vi "new_coating.vi"(0 "Coating":i32(listbox)) -> (1 "Recipe":string[](array[string]), 2 "Path Array":string[](array[string]))   [LabVIEW 2009]
panel:
  in  "Coating Name :":string
  in  "Recipe List":i32(listbox)
  in  "Move down":bool
  in  "Move up":bool
  out "error out":errorcluster
  in  "delete":bool
  in  "cancel":bool
  in  "ok":bool
  in  "Add Recipe":bool
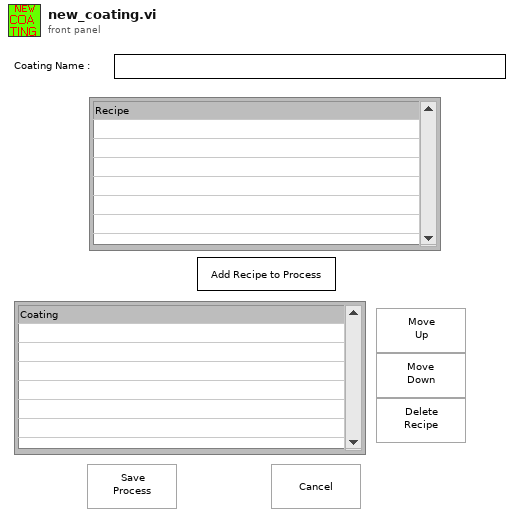
[diagram p1: front panel]
types:
  T1 = enum16{"open", "replace", "create", "open or create", "replace or create", "replace or create with confirmation"}
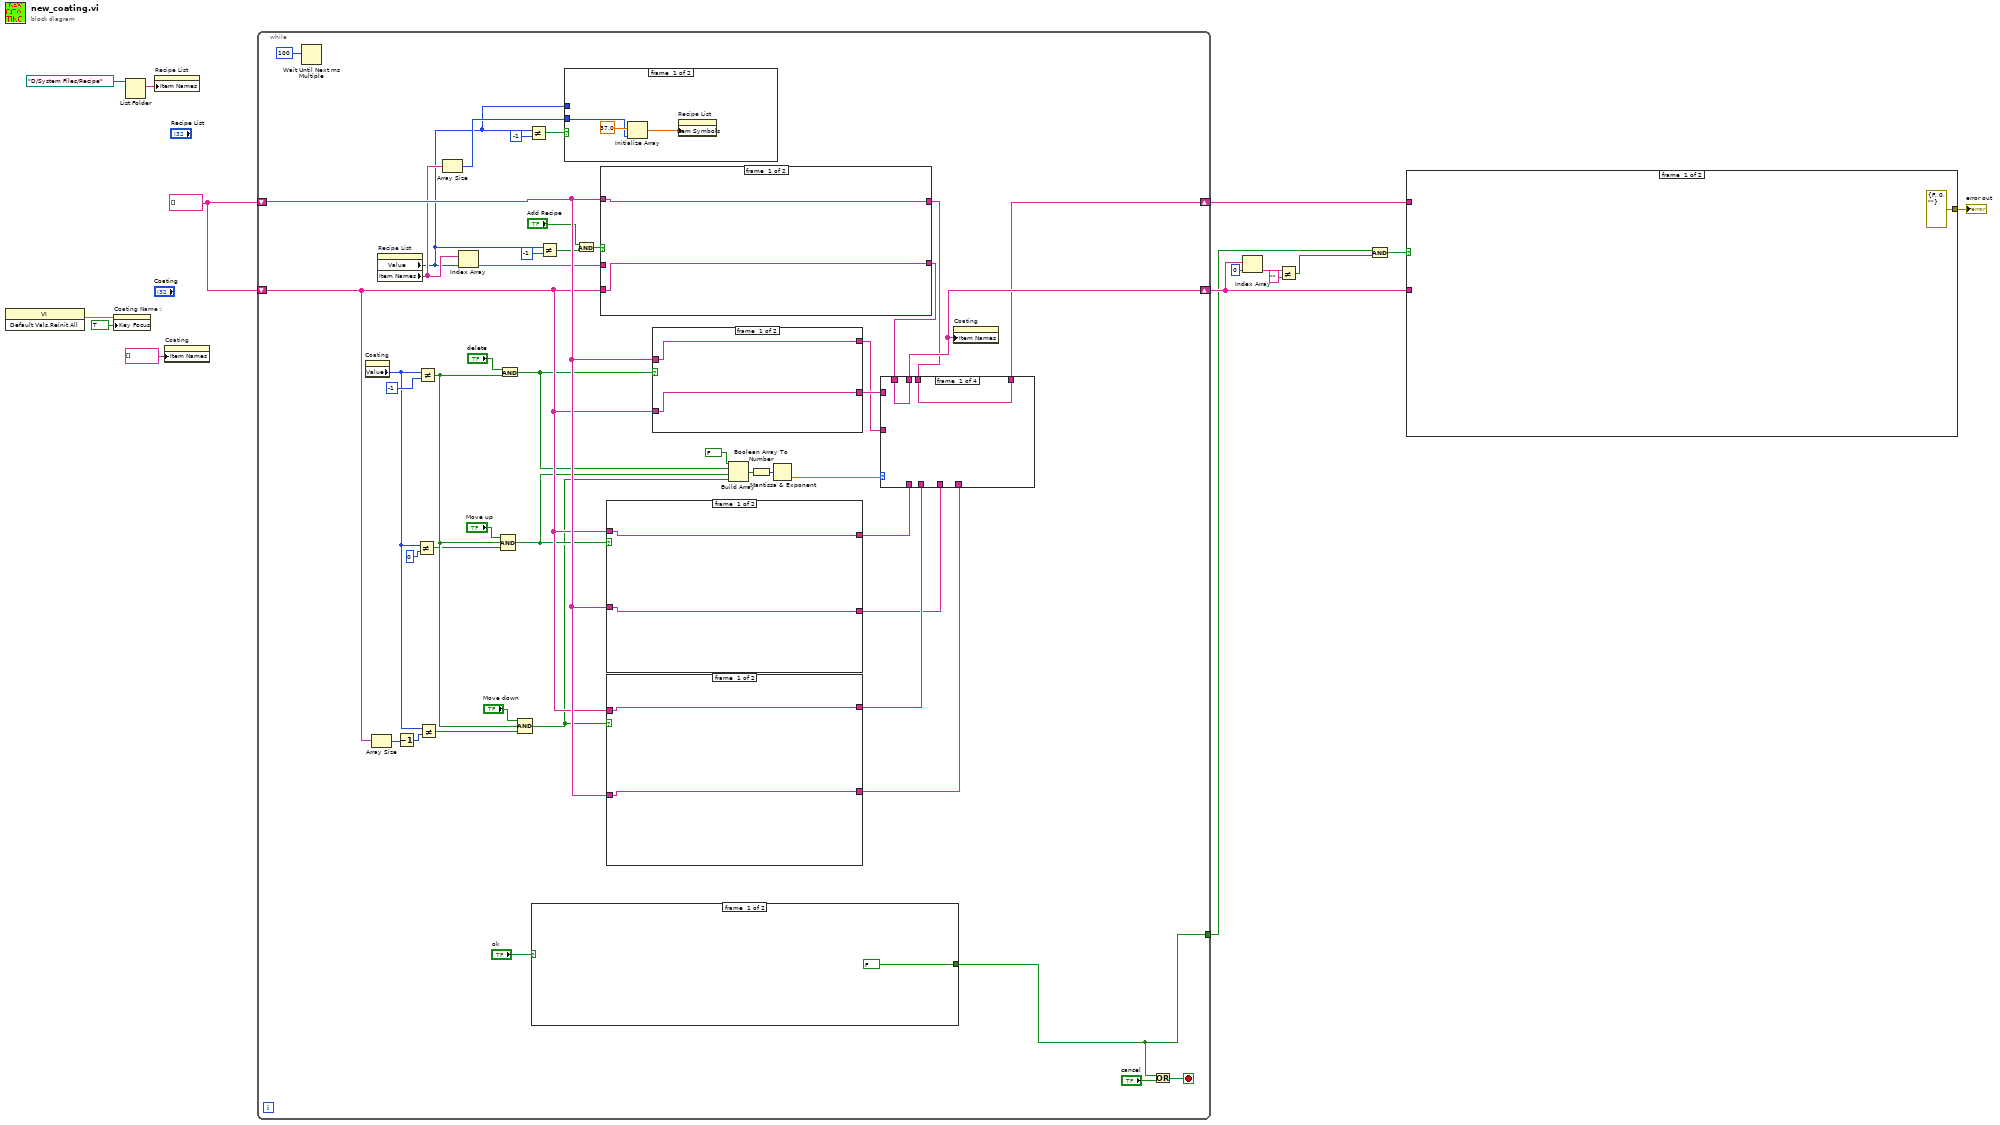
[diagram p0: block diagram]
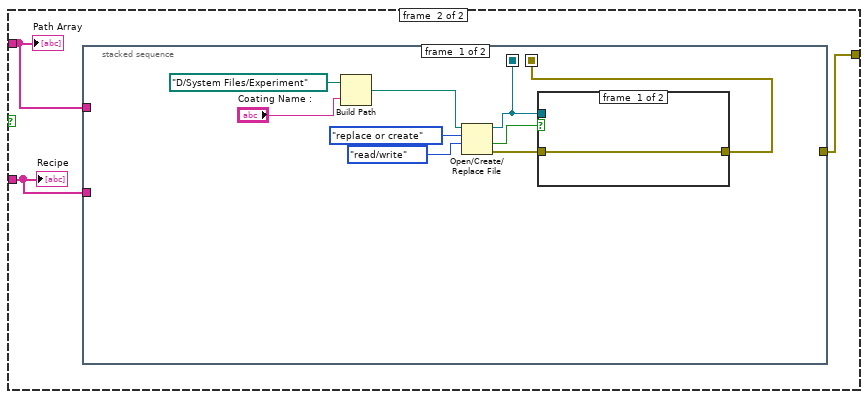
[diagram p2: hidden frame]
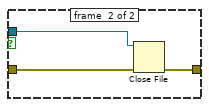
[diagram p3: hidden frame]
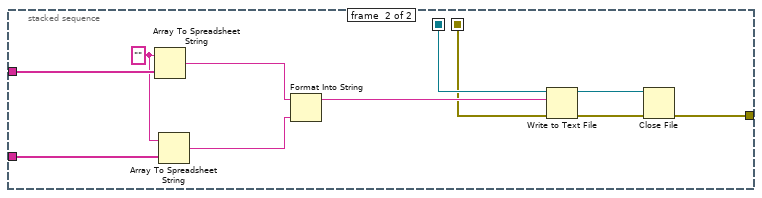
[diagram p4: hidden frame]
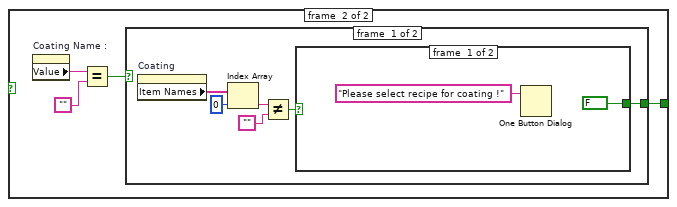
[diagram p5: hidden frame]
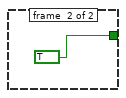
[diagram p6: hidden frame]
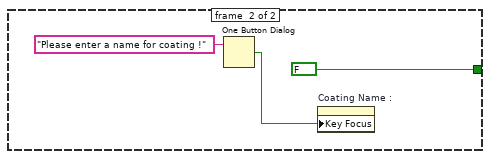
[diagram p7: hidden frame]
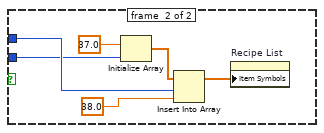
[diagram p8: hidden frame]
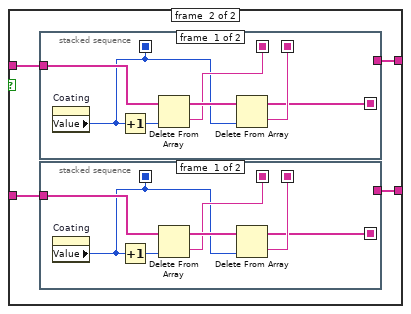
[diagram p12: hidden frame]
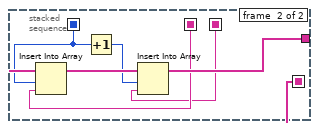
[diagram p13: hidden frame]
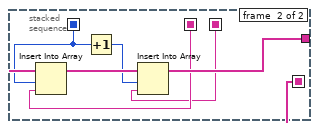
[diagram p14: hidden frame]
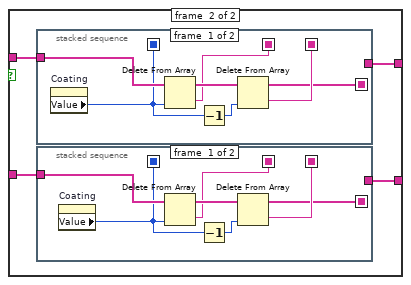
[diagram p15: hidden frame]
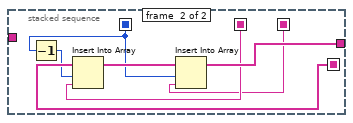
[diagram p16: hidden frame]
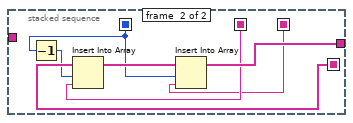
[diagram p17: hidden frame]
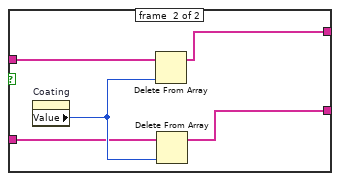
[diagram p18: hidden frame]
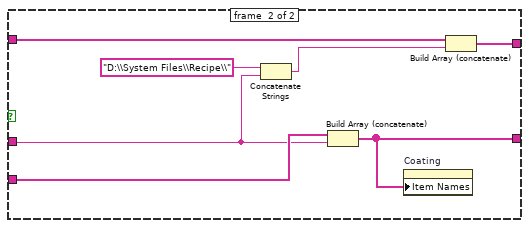
[diagram p19: hidden frame]
diagram:
  w15 = string[] []
  n1 = invoke class="VI" method="Default Vals.Reinit All"() -> (error out=w3:errorcluster)  [unwired: 3 in, 2 out]
  n2 = property on="Coating Name :" class="Str"(error in=w3, "Key Focus"=TRUE) -> ()  [unwired: 1 in, 2 out]
  n3 = List Folder(path=path "D:/System Files/Recipe") -> (filenames=w5:string[])  [unwired: 3 in, 3 out]
  n4 = property on="Recipe List" class="LstBox (strict)"("Item Names"=w5) -> ()  [unwired: 2 in, 2 out]
  n5 = property on="Coating" class="LstBox (strict)"("Item Names"=string[] []) -> ()  [unwired: 2 in, 2 out]
  n6 = while {
    shift-right: [w56] -> w14
    shift-left: w15 -> [w57]
    shift-right: [w58] -> w12
    shift-left: w15 -> [w55]
    tunnel: [w54] -> w1
    stop <- w59 stop-if-true
    n7 = Wait Until Next ms Multiple(millisecond multiple=100) -> ()  [unwired: 1 out]
    n8 = property on="Coating" class="LstBox (strict)"() -> ("Value"=w30:i32)  [unwired: 2 in, 2 out]
    n9 = Array Size(array=w55) -> (size(s)=w29:i32)
    n10 = property on="Recipe List" class="LstBox (strict)"() -> ("Value"=w18:i32, "Item Names"=w25:string[])  [unwired: 2 in, 2 out]
    n11 = Decrement(x=w29) -> (x-1=w28:i32)
    n12 = Not Equal?(x=w30, y=0) -> (x != y?=w32:bool)
    n13 = Not Equal?(x=w30, y=-1) -> (x != y?=w36:bool)
    n14 = Not Equal?(x=w30, y=w28) -> (x != y?=w31:bool)
    n15 = Array Size(array=w25) -> (size(s)=w23:i32)
    n16 = Index Array(array=w25, index=w18) -> (element=w27:string)
    n17 = And(x="delete", y=w36) -> (x .and. y?=w39:bool)
    n18 = Compound Arithmetic op=AND("Move up", w36, w32) -> (w37:bool)
    n19 = Compound Arithmetic op=AND("Move down", w36, w31) -> (w34:bool)
    n20 = Not Equal?(x=w18, y=-1) -> (x != y?=w24:bool)
    n21 = case shown="True" "ok" {
      tunnel: [FALSE w62] -> w54
      frame #0 {
      }
      frame #1 {
        n22 = property on="Coating Name :" class="Str"() -> ("Value"=w64:string)  [unwired: 2 in, 2 out]
        n23 = Equal?(x=w64, y="") -> (x = y?=w63:bool)
        n24 = case shown="True" w63 {
          tunnel: [w66 FALSE] -> w62
          frame #0 {
            n25 = property on="Coating" class="LstBox (strict)"() -> ("Item Names"=w69:string[])  [unwired: 2 in, 2 out]
            n26 = Index Array(array=w69, index=0) -> (element=w71:string)
            n27 = Not Equal?(x=w71, y="") -> (x != y?=w67:bool)
            n28 = case shown="False" w67 {
              tunnel: [FALSE TRUE] -> w66
              frame #0 {
                n29 = One Button Dialog(message="Please select recipe for coating !") -> ()  [unwired: 1 in, 1 out]
              }
              frame #1 {
              }
            }
          }
          frame #1 {
            n30 = One Button Dialog(message="Please enter a name for coating !") -> (true=w75:bool)  [unwired: 1 in]
            n31 = property on="Coating Name :" class="Str"("Key Focus"=w75) -> ()  [unwired: 2 in, 2 out]
          }
        }
      }
    }
    n32 = Not Equal?(x=w18, y=-1) -> (x != y?=w19:bool)
    n33 = case shown="False" w24 {
      tunnel: w18 -> [_ w83]
      tunnel: w23 -> [w79 w82]
      frame #0 {
        n34 = Initialize Array(37.0 ("element"), w79) -> (w78:dbl[])
        n35 = property on="Recipe List" class="LstBox (strict)"("Item Symbols"=w78) -> ()  [unwired: 2 in, 2 out]
      }
      frame #1 {
        n36 = Initialize Array(37.0 ("element"), w82) -> (w86:dbl[])
        n37 = Insert Into Array(array=w86, index=w83, new element=38.0 ("element")) -> (w81:dbl[])
        n38 = property on="Recipe List" class="LstBox (strict)"("Item Symbols"=w81) -> ()  [unwired: 2 in, 2 out]
      }
    }
    n39 = And(x="Add Recipe", y=w19) -> (x .and. y?=w21:bool)
    n40 = case shown="True" w21 {
      tunnel: [w171 w176] -> w45
      tunnel: [w170 w175] -> w46
      tunnel: w55 -> [w170 w178]
      tunnel: w57 -> [w171 w177]
      tunnel: w27 -> [_ w173]
      frame #0 {
      }
      frame #1 {
        n41 = Concatenate Strings("D:\\System Files\\Recipe\\" ("string"), w173) -> (w172:string)
        n42 = Build Array (concatenate)(w178, w173) -> (w175:string[])
        n43 = property on="Coating" class="LstBox (strict)"("Item Names"=w175) -> ()  [unwired: 2 in, 2 out]
        n44 = Build Array (concatenate)(w177, w172) -> (w176:string[])
      }
    }
    n45 = case shown="True" w37 {
      tunnel: w55 -> [w130 w134]
      tunnel: [w130 w133] -> w48
      tunnel: w57 -> [w129 w132]
      tunnel: [w129 w131] -> w44
      frame #0 {
      }
      frame #1 {
        n46 = stacked-sequence {
          seq-local: [w152 _] -> [_ w157]
          seq-local: [w151 _] -> [_ w156]
          seq-local: [w150 _] -> [_ w162]
          seq-local: [w149 _] -> [_ w159]
          tunnel: w134 -> [w155 _]
          tunnel: [_ w160] -> w133
          frame #0 {
            n47 = property on="Coating" class="LstBox (strict)"() -> ("Value"=w149:i32)  [unwired: 2 in, 2 out]
            n48 = Delete From Array(array=w155, index=w149) -> (deleted portion=w152:string, array with subset deleted=w154:string[])  [unwired: 1 in]
            n49 = Decrement(x=w149) -> (x-1=w153:i32)
            n50 = Delete From Array(array=w154, index=w153) -> (deleted portion=w151:string, array with subset deleted=w150:string[])  [unwired: 1 in]
          }
          frame #1 {
            n51 = Decrement(x=w159) -> (x-1=w158:i32)
            n52 = Insert Into Array(array=w162, index=w158, new element=w157) -> (w161:string[])
            n53 = Insert Into Array(array=w161, index=w159, new element=w156) -> (w160:string[])
          }
        }
        n54 = stacked-sequence {
          seq-local: [w138 _] -> [_ w143]
          seq-local: [w137 _] -> [_ w142]
          seq-local: [w136 _] -> [_ w148]
          seq-local: [w135 _] -> [_ w145]
          tunnel: w132 -> [w141 _]
          tunnel: [_ w146] -> w131
          frame #0 {
            n55 = property on="Coating" class="LstBox (strict)"() -> ("Value"=w135:i32)  [unwired: 2 in, 2 out]
            n56 = Delete From Array(array=w141, index=w135) -> (deleted portion=w138:string, array with subset deleted=w140:string[])  [unwired: 1 in]
            n57 = Decrement(x=w135) -> (x-1=w139:i32)
            n58 = Delete From Array(array=w140, index=w139) -> (deleted portion=w137:string, array with subset deleted=w136:string[])  [unwired: 1 in]
          }
          frame #1 {
            n59 = Decrement(x=w145) -> (x-1=w144:i32)
            n60 = Insert Into Array(array=w148, index=w144, new element=w143) -> (w147:string[])
            n61 = Insert Into Array(array=w147, index=w145, new element=w142) -> (w146:string[])
          }
        }
      }
    }
    n62 = case shown="True" w34 {
      tunnel: w55 -> [w96 w100]
      tunnel: [w96 w99] -> w47
      tunnel: w57 -> [w95 w98]
      tunnel: [w95 w97] -> w42
      frame #0 {
      }
      frame #1 {
        n63 = stacked-sequence {
          seq-local: [w117 _] -> [_ w125]
          seq-local: [w119 _] -> [_ w124]
          seq-local: [w118 _] -> [_ w128]
          seq-local: [w115 _] -> [_ w122]
          tunnel: w100 -> [w120 _]
          tunnel: [_ w127] -> w99
          frame #0 {
            n64 = property on="Coating" class="LstBox (strict)"() -> ("Value"=w115:i32)  [unwired: 2 in, 2 out]
            n65 = Increment(x=w115) -> (x+1=w116:i32)
            n66 = Delete From Array(array=w120, index=w116) -> (deleted portion=w117:string, array with subset deleted=w121:string[])  [unwired: 1 in]
            n67 = Delete From Array(array=w121, index=w115) -> (deleted portion=w119:string, array with subset deleted=w118:string[])  [unwired: 1 in]
          }
          frame #1 {
            n68 = Insert Into Array(array=w128, index=w122, new element=w125) -> (w126:string[])
            n69 = Increment(x=w122) -> (x+1=w123:i32)
            n70 = Insert Into Array(array=w126, index=w123, new element=w124) -> (w127:string[])
          }
        }
        n71 = stacked-sequence {
          seq-local: [w103 _] -> [_ w111]
          seq-local: [w105 _] -> [_ w110]
          seq-local: [w104 _] -> [_ w114]
          seq-local: [w101 _] -> [_ w108]
          tunnel: w98 -> [w106 _]
          tunnel: [_ w113] -> w97
          frame #0 {
            n72 = property on="Coating" class="LstBox (strict)"() -> ("Value"=w101:i32)  [unwired: 2 in, 2 out]
            n73 = Increment(x=w101) -> (x+1=w102:i32)
            n74 = Delete From Array(array=w106, index=w102) -> (deleted portion=w103:string, array with subset deleted=w107:string[])  [unwired: 1 in]
            n75 = Delete From Array(array=w107, index=w101) -> (deleted portion=w105:string, array with subset deleted=w104:string[])  [unwired: 1 in]
          }
          frame #1 {
            n76 = Insert Into Array(array=w114, index=w108, new element=w111) -> (w112:string[])
            n77 = Increment(x=w108) -> (x+1=w109:i32)
            n78 = Insert Into Array(array=w112, index=w109, new element=w110) -> (w113:string[])
          }
        }
      }
    }
    n79 = case shown="True" w39 {
      tunnel: w57 -> [w163 w169]
      tunnel: w55 -> [w164 w167]
      tunnel: [w164 w166] -> w49
      tunnel: [w163 w165] -> w43
      frame #0 {
      }
      frame #1 {
        n80 = property on="Coating" class="LstBox (strict)"() -> ("Value"=w168:i32)  [unwired: 2 in, 2 out]
        n81 = Delete From Array(array=w169, index=w168) -> (array with subset deleted=w165:string[])  [unwired: 1 in, 1 out]
        n82 = Delete From Array(array=w167, index=w168) -> (array with subset deleted=w166:string[])  [unwired: 1 in, 1 out]
      }
    }
    n83 = Build Array(FALSE, w39, w37, w34) -> (w51:bool[])
    n84 = Boolean Array To Number(Boolean array=w51) -> (number=w52:u32)
    n85 = Mantissa & Exponent(0:w52) -> (2:w50:dbl)  [unwired: 1 out]
    n86 = case shown="0, Default" w50 {
      tunnel: w49 -> [_ w90 _ _]
      tunnel: [w88 w90 w92 w94] -> w58
      tunnel: w48 -> [_ _ w92 _]
      tunnel: w47 -> [_ _ _ w94]
      tunnel: w46 -> [w88 _ _ _]
      tunnel: w45 -> [w87 _ _ _]
      tunnel: [w87 w89 w91 w93] -> w56
      tunnel: w44 -> [_ _ w91 _]
      tunnel: w43 -> [_ w89 _ _]
      tunnel: w42 -> [_ _ _ w93]
      frame #0 {
      }
      frame #1 {
      }
      frame #2 {
      }
      frame #3 {
      }
    }
    n87 = property on="Coating" class="LstBox (strict)"("Item Names"=w58) -> ()  [unwired: 2 in, 2 out]
    n88 = Or(x=w54, y="cancel") -> (x .or. y?=w59:bool)
  }
  n89 = Index Array(array=w12, index=0) -> (element=w10:string)
  n90 = Not Equal?(x=w10, y="") -> (x != y?=w8:bool)
  n91 = Compound Arithmetic op=AND(w1, w8) -> (w7:bool)
  n92 = case shown="True" w7 {
    tunnel: w14 -> [_ w181]
    tunnel: w12 -> [_ w182]
    tunnel: [errorcluster {"status"=FALSE, "code"=0, "source"=""} ("error out") w180] -> w6
    frame #0 {
    }
    frame #1 {
      n93 = stacked-sequence {
        seq-local: [w188 _] -> [_ w201]
        seq-local: [w186 _] -> [_ w197]
        tunnel: w181 -> [_ w206]
        tunnel: w182 -> [_ w205]
        tunnel: [_ w196] -> w180
        frame #0 {
          n94 = Build Path(base path=path "D:/System Files/Experiment" ("start path"), name or relative path="Coating Name :") -> (appended path=w183:path)
          n95 = Open/Create/Replace File(file path (use dialog)=w183, operation (0:open)=T1."replace or create", access (0:read/write)=enum16{"read/write", "read-only", "write-only"}."read/write") -> (refnum out=w188:refnum<file>, cancelled=w190:bool, error out=w187:errorcluster)  [unwired: 3 in]
          n96 = case shown="True" w190 {
            tunnel: w188 -> [_ w195]
            tunnel: w187 -> [w192 w194]
            tunnel: [w192 w193] -> w186
            frame #0 {
            }
            frame #1 {
              n97 = Close File(refnum=w195, error in=w194) -> (error out=w193:errorcluster)  [unwired: 1 out]
            }
          }
        }
        frame #1 {
          w200 = "" ("format string")
          n98 = Array To Spreadsheet String(array=w206, 3:w200) -> (spreadsheet string=w204:string)  [unwired: 1 in]
          n99 = Array To Spreadsheet String(array=w205, 3:w200) -> (spreadsheet string=w203:string)  [unwired: 1 in]
          n100 = Format Into String(initial string=w204, w203) -> (resulting string=w202:string)  [unwired: 2 in, 1 out]
          n101 = Write to Text File(file (use dialog)=w201, text=w202, error in=w197) -> (refnum out=w198:refnum<file>, error out=w199:errorcluster)  [unwired: 1 in, 1 out]
          n102 = Close File(refnum=w198, error in=w199) -> (error out=w196:errorcluster)  [unwired: 1 out]
        }
      }
      "Path Array" <- w181
      "Recipe" <- w182
    }
  }
  "error out" <- w6
